vi "Client 1 - Copy.vi"() -> ()   [LabVIEW 2017]
uses:
  <vilib>/Analysis/Matrix/NI_Matrix.lvlib
  <vilib>/Analysis/Matrix/Numeric/Multiply/Multiply - RM,RM.vi
  <vilib>/Analysis/Matrix/Datatypes/RealMatrix.ctl
panel:
  out "M1 x M2":T1
  in  "Matrix 1":T1
  in  "Matrix 2":T1
  out "bytes written":i32
  out "data string":string
  in  "stop":bool
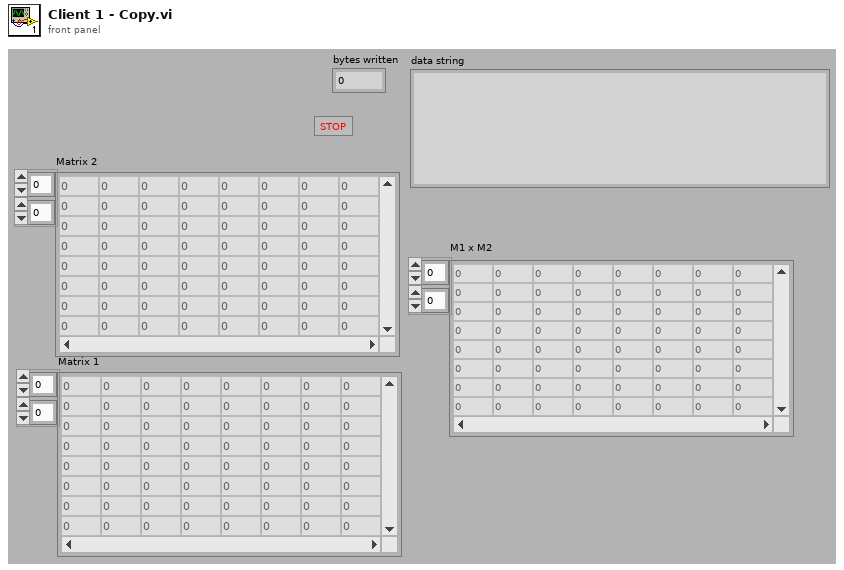
[diagram p1: front panel]
types:
  T1 = typedef "NI_Matrix.lvlib/RealMatrix.ctl" = dbl[][]
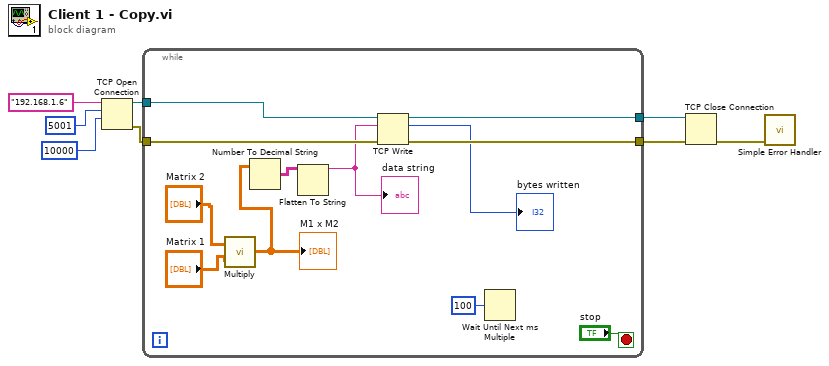
[diagram p0: block diagram]
diagram:
  n1 = TCP Open Connection(address="192.168.1.6", remote port or service name=u16 5001, timeout ms (60000)=10000) -> (connection ID=w5:refnum<k5>, error out=w4:errorcluster)  [unwired: 2 in]
  n2 = while {
    tunnel: w5 -> [w19]
    tunnel: w4 -> [w18]
    tunnel: [w17] -> w2
    tunnel: [w16] -> w1
    stop <- "stop" stop-if-true
    n3 = call-poly <vilib>:"Multiply.vi"("Real Matrix B"="Matrix 1", "Real Matrix A"="Matrix 2") -> ("A * B"=w10:T1)
    "M1 x M2" <- w10
    n4 = Number To Decimal String(number=w10) -> (decimal integer string=w11:string[][])  [unwired: 1 in]
    n5 = Flatten To String(anything=w11) -> (data string=w12:string)  [unwired: 3 in, 2 out]
    "data string" <- w12
    n6 = TCP Write(connection ID=w19, data in=w12, error in (no error)=w18) -> (connection ID out=w17:refnum<k5>, bytes written=→"bytes written":i32, error out=w16:errorcluster)  [unwired: 1 in]
    n7 = Wait Until Next ms Multiple(millisecond multiple=u32 100) -> ()  [unwired: 1 out]
  }
  n8 = TCP Close Connection(connection ID=w2, error in (no error)=w1) -> (error out=w3:errorcluster)  [unwired: 1 in, 1 out]
  n9 = call <vilib>:"Simple Error Handler.vi"("error in (no error)"=w3) -> ()  [unwired: 4 in, 5 out]
